vi "lua_call.vi"(8 "error in":errorcluster, 9 "nresults":i32, 10 "nargs":i32, 11 "lua_State *L":u64) -> (0 "error out":errorcluster)   [LabVIEW 2011]
doc: "void lua_call (lua_State *L, int nargs, int nresults);\nCalls a function. \n#define lua_call(L,n,r) lua_callk(L, (n), (r), 0, NULL)\n\nTo call a function you must use the following protocol: first, the function to be called is pushed onto the stack; then, the arguments to the function are pushed in direct order; that is, the first argument is pushed first. Finally you call lua_call; nargs is the number of arguments that you pushed onto the stack. All arguments and the function value are popped from the stack when the function is called. The function results are pushed onto the stack when the function returns. The number of results is adjusted to nresults, unless nresults is LUA_MULTRET. In this case, all results from the function are pushed. Lua takes care that the returned values fit into the stack space. The function results are pushed onto the stack in direct order (the first result is pushed first), so that after the call the last result is on the top of the stack. \n\nAny error inside the called function is propagated upwards (with a longjmp). \n\nThe following example shows how the host program can do the equivalent to this Lua code: \n\n a = f(\"how\", t.x, 14)\n\nHere it is in C: \n\n lua_getglobal(L, \"f\"); /* function to be called */\n lua_pushstring(L, \"how\"); /* 1st argument */\n lua_getglobal(L, \"t\"); /* table to be indexed */\n lua_getfield(L, -1, \"x\"); /* push result of t.x (2nd arg) */\n lua_remove(L, -2); /* remove 't' from the stack */\n lua_pushinteger(L, 14); /* 3rd argument */c\n lua_call(L, 3, 1); /* call 'f' with 3 arguments and 1 result */\n lua_setglobal(L, \"a\"); /* set global 'a' */\n\nNote that the code above is \"balanced\": at its end, the stack is back to its original configuration. This is considered good programming practice."
uses:
  lua5.1.dll
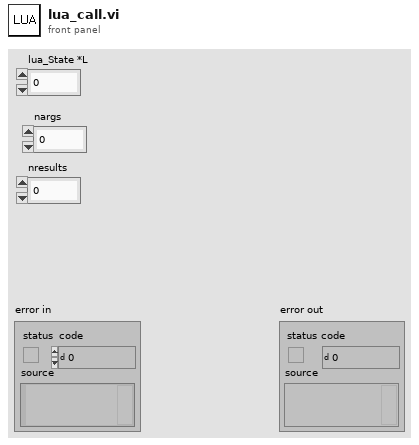
[diagram p1: front panel]
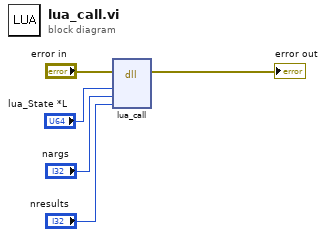
[diagram p0: block diagram]
diagram:
  n1 = dll-call lib="lua5.1.dll" fn="lua_call"(error in="error in", "lua_State *L"="lua_State *L", "nargs"="nargs", "nresults"="nresults") -> (error out=→"error out":errorcluster)  [unwired: 6 in, 1 out]
